vi "Get UI Control Value.vi"(8 "error in (no error)":errorcluster, 10 "VI Ref":refnum<vi>, 11 "Boolean Parameter in":refnum<class "String Parameter.lvclass">) -> (0 "error out":errorcluster, 3 "Boolean Parameter out":refnum<class "String Parameter.lvclass">)   [LabVIEW 2016, in "CD Parameter Manager API.lvlib" / "String Parameter.lvclass"]
uses:
  String Parameter.lvclass
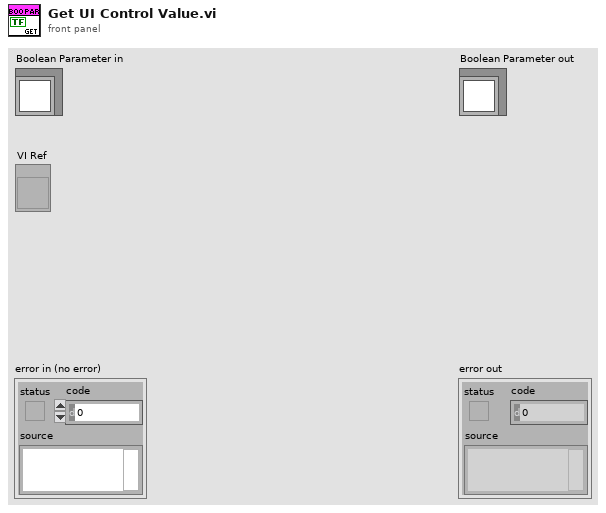
[diagram p1: front panel]
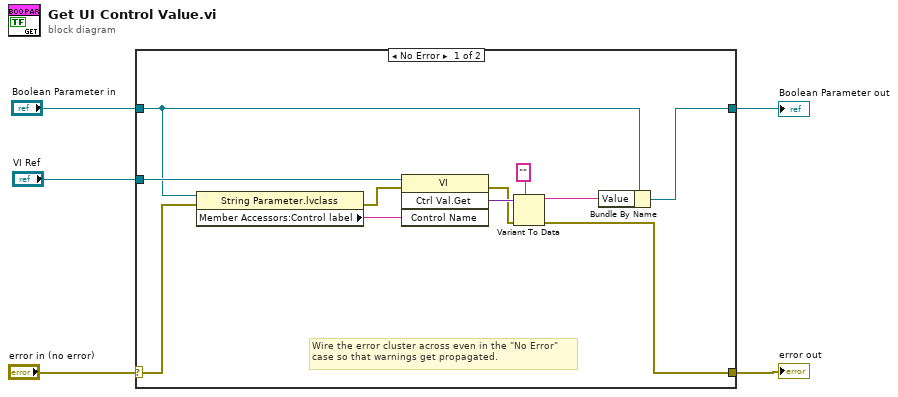
[diagram p0: block diagram]
diagram:
  n1 = case shown="No Error" "error in (no error)" {
    selector: "error in (no error)" -> [w11 w18]
    tunnel: [w8 w18] -> w4
    tunnel: [w15 w17] -> w5
    tunnel: "Boolean Parameter in" -> [w13 w17]
    tunnel: "VI Ref" -> [w16 _]
    frame No Error {
      # "Wire the error cluster across even in the \"No Error\"\ncase so that warnings get propagated."
      n2 = property class="String Parameter.lvclass"(reference=w13, error in=w11) -> (error out=w10:errorcluster, "Member Accessors:Control label"=w12:string)  [unwired: 1 out]
      n3 = invoke class="VI" method="Ctrl Val.Get"(reference=w16, error in=w10, "Control Name"=w12) -> (error out=w9:errorcluster, "Get Control Value Variant"=w14:variant)  [unwired: 1 in, 2 out]
      n4 = Variant To Data(error in=w9, type="" ("Value"), Variant=w14) -> (data=w6:string, error out=w8:errorcluster)
      n5 = Bundle By Name(cluster=w13, "Value"=w6) -> (w15:refnum<class "String Parameter.lvclass">)
    }
    frame Error {
    }
  }
  "error out" <- w4
  "Boolean Parameter out" <- w5
